vi "Dialog_ZeroAdjust.vi"() -> (6 "OK":bool)   [LabVIEW 2015]
panel:
  in  "Cancel":bool
  in  "stop":bool
  # "Zero adjustment\nCover sensor and press OK"
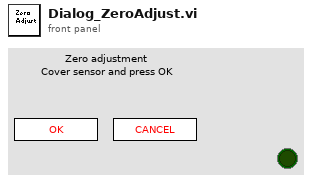
[diagram p1: front panel]
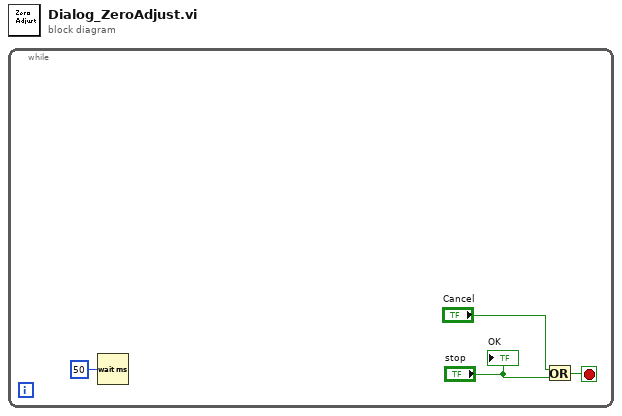
[diagram p0: block diagram]
diagram:
  n1 = while {
    stop <- w3 stop-if-true
    n2 = Wait (ms)(milliseconds to wait=u32 50) -> ()  [unwired: 1 out]
    n3 = Or(x="Cancel", y="stop") -> (x .or. y?=w3:bool)
    "OK" <- "stop"
  }
